vi "Update Progess Bar.vi"(8 "error in (no error)":errorcluster, 11 "Progess Bar":u8 max=100) -> (0 "error out":errorcluster)   [LabVIEW 2019, in "Status.lvlib"]
uses:
  Status.lvlib
  Message Queue/State Name.ctl
  Message Queue/Reference Queue.vi
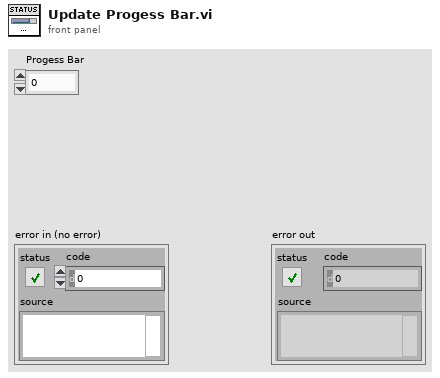
[diagram p1: front panel]
types:
  T1 = typedef "Status.lvlib/State Name.ctl" = enum16{"Initialize", "Update Progress Bar", "Update Status Bar", "Set Cursor Busy", "Unset Cursor Busy", "Error", "Default", "Exit"}
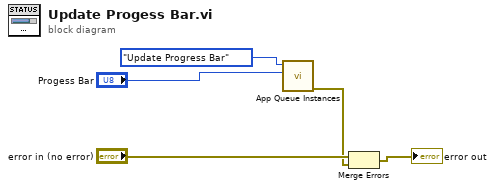
[diagram p0: block diagram]
diagram:
  n1 = call-poly "App Queue Instances.vi"("Message Data"="Progess Bar", "Tasks"=State_Name."Update Progress Bar" ("States")) -> ("error out"=w3:errorcluster)  [unwired: 9 in]
  n2 = Merge Errors("error in (no error)", w3) -> (→"error out":errorcluster)
